vi "PC_Pub_imgFile getDataInfo.vi"(7 "getTitle":string[](array[string])=["Title", "Description", "Version"], 8 "error in (no error)":errorcluster, 11 "dataString":string) -> (0 "error out":errorcluster, 3 "getValue":string[](array[string]))   [LabVIEW 2018, in "PC_Pub_imgFile.lvclass"]
uses:
  PC_Pub_imgFile.lvclass
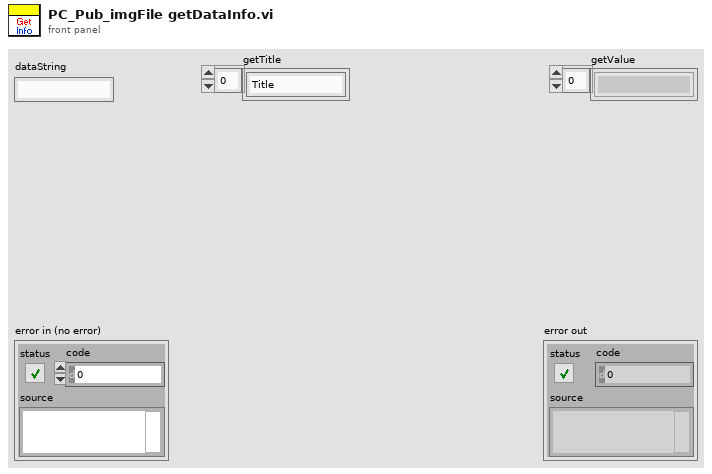
[diagram p1: front panel]
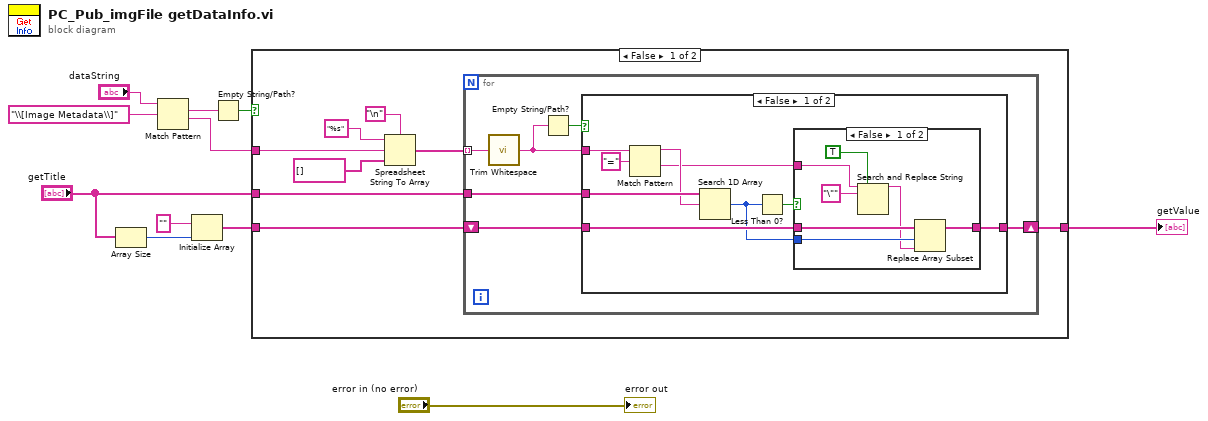
[diagram p0: block diagram]
diagram:
  n1 = Array Size(array="getTitle") -> (size(s)=w4:i32)
  n2 = Match Pattern(string="dataString", regular expression="\\[Image Metadata\\]") -> (match substring=w8:string, after substring=w9:string)  [unwired: 1 in, 2 out]
  n3 = Initialize Array("", w4) -> (w2:string[])
  n4 = Empty String/Path?(string/path=w8) -> (empty?=w7:bool)
  n5 = case shown="False" w7 {
    tunnel: w9 -> [w16 _]
    tunnel: "getTitle" -> [w14 _]
    tunnel: [w13 w44] -> w6
    tunnel: w2 -> [w12 w44]
    frame False {
      n6 = Spreadsheet String To Array(delimiter (Tab)="\n", format string="%s", spreadsheet string=w16, array type (2D Dbl)=string[] []) -> (array=w15:string[])
      n7 = for {
        tunnel: w15 -> [w25] mode=indexing
        shift-right: [w20] -> w13
        shift-left: w12 -> [w21]
        tunnel: w14 -> [w22]
        n8 = call <vilib>:"Trim Whitespace.vi"("string"=w25) -> ("trimmed string"=w23:string)  [unwired: 1 in]
        n9 = Empty String/Path?(string/path=w23) -> (empty?=w24:bool)
        n10 = case shown="False" w24 {
          tunnel: w23 -> [w33 _]
          tunnel: w22 -> [w32 _]
          tunnel: w21 -> [w29 w43]
          tunnel: [w26 w43] -> w20
          frame False {
            n11 = Match Pattern(string=w33, regular expression="=") -> (before substring=w31:string, after substring=w28:string)  [unwired: 1 in, 2 out]
            n12 = Search 1D Array(1D array=w32, element=w31) -> (index of element=w27:i32)  [unwired: 1 in]
            n13 = Less Than 0?(x=w27) -> (x < 0?=w30:bool)
            n14 = case shown="False" w30 {
              tunnel: w29 -> [w41 w42]
              tunnel: w28 -> [w36 _]
              tunnel: w27 -> [w40 _]
              tunnel: [w39 w42] -> w26
              frame False {
                n15 = Search and Replace String(replace all?=TRUE ("replace all? (F)"), input string=w36, search string="\"") -> (result string=w35:string)  [unwired: 5 in, 3 out]
                n16 = Replace Array Subset(array=w41, new element=w35, index=w40) -> (w39:string[])
              }
              frame True {
              }
            }
          }
          frame True {
          }
        }
      }
    }
    frame True {
    }
  }
  "getValue" <- w6
  "error out" <- "error in (no error)"
